vi "Reinitialize.vi"(8 "error in (no error)":errorcluster, 11 "ProPar in":refnum<class "PL Bronkhorst ProPar.lvclass">) -> (0 "error out":errorcluster, 3 "ProPar out":refnum<class "PL Bronkhorst ProPar.lvclass">)   [LabVIEW 2015, in "PL Bronkhorst ProPar.lvclass"]
doc: "Reinitializes connection to device based on previously specified settings."
uses:
  PL Bronkhorst ProPar.lvclass
  PL Bronkhorst ProPar.lvclass/PL Bronkhorst ProPar.ctl
  <vilib>/Instr/_visa.llb/VISA Configure Serial Port (Instr).vi
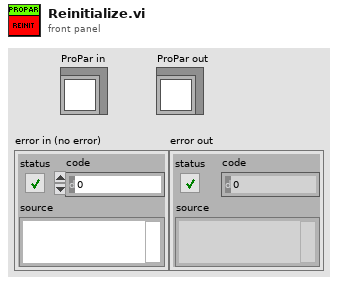
[diagram p1: front panel]
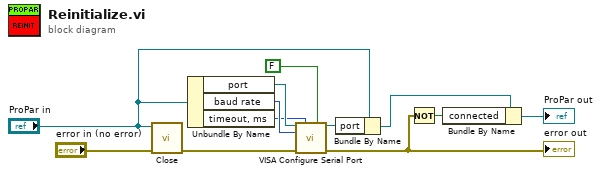
[diagram p0: block diagram]
diagram:
  n1 = call "Close.vi"("error in (no error)"="error in (no error)", "ProPar in"="ProPar in") -> ("error out"=w5:errorcluster)  [unwired: 9 in]
  n2 = Unbundle By Name("ProPar in") -> ("port"=w6:refnum<visa-resource-name>, "baud rate"=w7:u32, "timeout, ms"=w1:u32)
  n3 = call-poly "VISA Configure Serial Port"("VISA resource name"=w6, "timeout (10sec)"=w1, "Enable Termination\nChar (T)"=FALSE ("Enable Termination\nChar (T)"), "baud rate (9600)"=w7, "error in (no error)"=w5) -> ("VISA resource name out"=w4:refnum<visa-resource-name>, "error out"=w3:errorcluster)  [unwired: 9 in]
  "error out" <- w3
  n4 = Bundle By Name(cluster="ProPar in", "port"=w4) -> (w11:refnum<class "PL Bronkhorst ProPar.lvclass">)
  n5 = Not(x=w3) -> (.not. x?=w10:bool)
  n6 = Bundle By Name(cluster=w11, "connected"=w10) -> (→"ProPar out":refnum<class "PL Bronkhorst ProPar.lvclass">)
